vi "AIT 664 - Add Multiple Bit Channels.vi"(8 "error in (no error)":errorcluster, 11 "Node Ptr":u64 format="%.0x") -> (0 "error out":errorcluster)   [LabVIEW 2014, in "AIT 664 Custom Device.lvlib"]
doc: "Add multiple bit channels to port."
uses:
  AIT 664 Custom Device.lvlib
  <vilib>/NI Veristand/Custom Device API/Custom Device Channel.ctl
  <vilib>/NI Veristand/Custom Device API/Custom Device Channel Type.ctl
  Controls/664 -Param.ctl
  Controls and Global/Global.vi
  <vilib>/NI Veristand/Custom Device API/Get Item Property (U32 Array).vi
  <vilib>/NI Veristand/Custom Device API/Get Item Property (Boolean).vi
  <vilib>/NI Veristand/Custom Device API/Custom Device API.lvlib
panel:
  in  "Cancel":bool
  in  "OK":bool
  in  "Number of Bits":i32=8 min=1 max=32 step=1
  in  "Start Bit":i32 min=0 max=31 step=1
  in  "Start Word":i32=1 min=1 max=31 step=1
  # "Add Multiple Bit Channels"
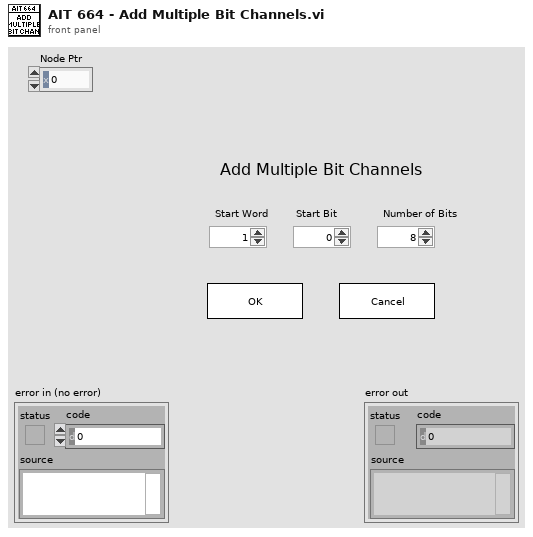
[diagram p1: front panel]
types:
  T1 = enum32{"Invalid", "Standard", "Closed", "Hidden", "Minimized", "Maximized"}
  T2 = typedef "Custom Device API.lvlib/Custom Device Channel Type.ctl" = enum16{"Input", "Output"}
  T3 = typedef "Custom Device API.lvlib/Custom Device Channel.ctl" = cluster{"Type":T2, "Units":string, "Default Value":dbl, "Faultable":bool, "Scalable":bool}
  T4 = typedef "AIT 664 Custom Device.lvlib/664 -Param.ctl" = cluster{"name":string, "firstByte":i32, "startBit":i32, "numberBits":i32, "scaleFactor":dbl, "scaleOffset":dbl, "signed":bool}
  T5 = typedef "Custom Device API.lvlib/Custom Device Item Ref.ctl" = u64
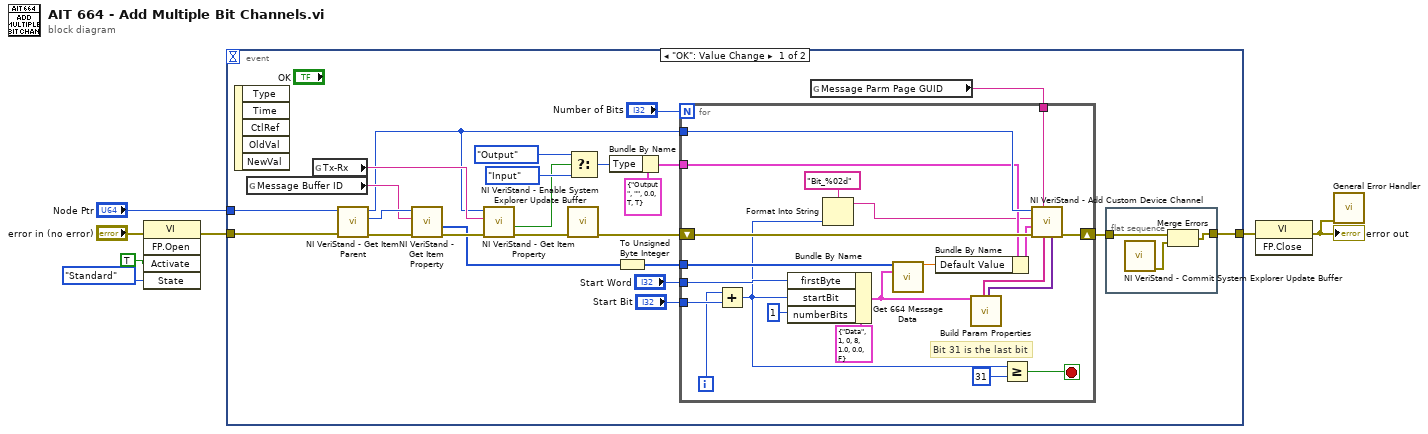
[diagram p0: block diagram]
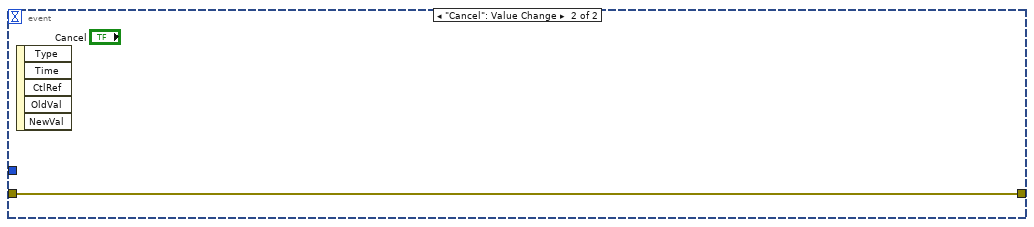
[diagram p2: hidden frame]
diagram:
  n1 = invoke class="VI" method="FP.Open"(error in="error in (no error)", "Activate"=TRUE ("Activate?"), "State"=T1."Standard") -> (error out=w3:errorcluster)  [unwired: 2 in, 4 out]
  n2 = event shown="[0] \"OK\": Value Change" {
    selector: _ -> [_ _]
    dyn-events: _ -> [_ _]
    timeout: _ -> [_ _]
    tunnel: [w12 w56] -> w7
    tunnel: w3 -> [w10 w56]
    tunnel: "Node Ptr" -> [w9 _]
    event "OK": Value Change {
      n3 = event-data() -> ()  [unwired: 1 in, 5 out]
      n4 = global read "Global.vi" "Message Buffer ID"() -> (w22:string)
      n5 = global read "Global.vi" "Tx-Rx"() -> (w21:string)
      n6 = call <vilib>:"NI VeriStand - Get Item Parent.vi"("error in (no error)"=w10, "Item Ref in"=w9) -> ("error out"=w24:errorcluster, "Parent Ref"=w23:T5, "Item Ref out"=w8:T5)  [unwired: 6 in, 1 out]
      n7 = call-poly <vilib>:"NI VeriStand - Get Item Property.vi"("error in (no error)"=w24, "Property Name"=w22, "Item Ref in"=w23) -> ("error out"=w20:errorcluster, "Value"=w18:u32[])  [unwired: 5 in, 2 out]
      n8 = call-poly <vilib>:"NI VeriStand - Get Item Property.vi"("error in (no error)"=w20, "Property Name"=w21, "Item Ref in"=w8) -> ("error out"=w16:errorcluster, "Value"=w15:bool)  [unwired: 5 in, 2 out]
      n9 = call <vilib>:"NI VeriStand - Enable System Explorer Update Buffer.vi"("error in (no error)"=w16) -> ("error out"=w26:errorcluster)  [unwired: 10 in]
      n10 = Select(t=Custom_Device_Channel_Type."Output" ("Type"), s=w15, f=Custom_Device_Channel_Type."Input" ("Type")) -> (s? t:f=w29:T2)
      n11 = Bundle By Name(cluster=T3 {"Type"=enum."Output", "Units"="", "Default Value"=0.0, "Faultable"=TRUE, "Scalable"=TRUE} ("Channel"), "Type"=w29) -> (w28:T3)
      n12 = To Unsigned Byte Integer(number=w18) -> (unsigned 8bit integer=w17:u8[])
      n13 = global read "Global.vi" "Message Parm Page GUID"() -> (w27:string)
      n14 = for {
        N: "Number of Bits" -> [_]
        shift-right: [w54] -> w25
        shift-left: w26 -> [w55]
        tunnel: w8 -> [w53]
        tunnel: w28 -> [w52]
        tunnel: w27 -> [w51]
        tunnel: "Start Word" -> [w45]
        tunnel: w17 -> [w49]
        tunnel: "Start Bit" -> [w41]
        i -> [w36]
        stop <- w39 stop-if-true
        # "Bit 31 is the last bit"
        n15 = Add(x=w36, y=w41) -> (x+y=w35:i32)
        n16 = Bundle By Name(cluster=T4 {"name"="Data", "firstByte"=1, "startBit"=0, "numberBits"=8, "scaleFactor"=1.0, "scaleOffset"=0.0, "signed"=FALSE} ("1553 Parameter"), "firstByte"=w45, "startBit"=w35, "numberBits"=1) -> (w44:T4)
        n17 = Format Into String(format string="Bit_%02d" ("string"), w35) -> (resulting string=w37:string)  [unwired: 2 in, 1 out]
        n18 = call "Get 664 Message Data.vi"("MSG DATA"=w49, "664 Parameter"=w44) -> ("Value"=w48:dbl)  [unwired: 12 in, 1 out]
        n19 = Bundle By Name(cluster=w52, "Default Value"=w48) -> (w50:T3)
        n20 = call "Build Param Properties.vi"("Parameter"=w44) -> ("Prop Names"=w43:string[], "Prop Values"=w42:variant[])  [unwired: 10 in, 7 out]
        n21 = Greater Or Equal?(x=w35, y=31) -> (x >= y?=w39:bool)
        n22 = call <vilib>:"NI VeriStand - Add Custom Device Channel.vi"("Property Values"=w42, "Property names"=w43, "GUID (Default Channel)"=w51, "error in (no error)"=w55, "Channel"=w50, "Channel Name"=w37, "Parent Ref in"=w53) -> ("error out"=w54:errorcluster)  [unwired: 1 in, 3 out]
      }
      n23 = flat-sequence {
        tunnel: w25 -> [w34]
        tunnel: [w32] -> w12
        frame #0 {
          n24 = call <vilib>:"NI VeriStand - Commit System Explorer Update Buffer.vi"() -> ("error out"=w33:errorcluster)  [unwired: 11 in]
          n25 = Merge Errors(w34, w33) -> (w32:errorcluster)
        }
      }
    }
    event "Cancel": Value Change {
      n26 = event-data() -> ()  [unwired: 1 in, 5 out]
    }
  }
  n27 = invoke class="VI" method="FP.Close"(error in=w7) -> (error out=w6:errorcluster)  [unwired: 2 in, 2 out]
  "error out" <- w6
  n28 = call <vilib>:"General Error Handler.vi"("error in (no error)"=w6) -> ()  [unwired: 10 in, 5 out]
